vi "SimulateData.vi"(7 "DAQ":T1={"Data"={"Live"={"t0"=timestamp(0 s since 1904-01-01), "dt"=1.0, "Y"=[]}, "Accumulated"={"t0"=timestamp(0 s since 1904-01-01), "dt"=1.0, "Y"=[]}, "Averaged"={"t0"=timestamp(0 s since 1904-01-01), "dt"=1.0, "Y"=[]}, "data array"=[], "live time array"=[], "Live (decimated)"={"t0"=timestamp(0 s since 1904-01-01), "dt"=1.0, "Y"=[]}}, "Config"={"Input Config"=0, "Card"=enum."USB-6211", "100% Reflectance Standard (V)"=0.0, "Input Channel"="", "Average number of points"=0.0, "Trigger Level (V)"=0.0, "Rate (Hz)"=0, "End Time (s)"=0.0}, "Indicators"={"Final number of points"=0.0, "Number of samples"=0.0, "dt"=0.0, "Shots"=10, "Shot counter"=10, "Test counter"=10, "Background level (V)"=0.0, "DAQ task"="", "timestamp of data"=timestamp(0 s since 1904-01-01), "Test Type"=enum."A-Test"}} {"Config"."Input Config" items=["default"=-1, "RSE"=10083, "NRSE"=10078, "Differential"=10106, "Pseudodifferential"=12529]}, 8 "error in (no error)":errorcluster) -> (0 "error out":errorcluster, 5 "DAQ out":T1={"Data"={"Live"={"t0"=timestamp(0 s since 1904-01-01), "dt"=1.0, "Y"=[]}, "Accumulated"={"t0"=timestamp(0 s since 1904-01-01), "dt"=1.0, "Y"=[]}, "Averaged"={"t0"=timestamp(0 s since 1904-01-01), "dt"=1.0, "Y"=[]}, "data array"=[], "live time array"=[], "Live (decimated)"={"t0"=timestamp(0 s since 1904-01-01), "dt"=1.0, "Y"=[]}}, "Config"={"Input Config"=0, "Card"=enum."USB-6211", "100% Reflectance Standard (V)"=0.0, "Input Channel"="", "Average number of points"=0.0, "Trigger Level (V)"=0.0, "Rate (Hz)"=0, "End Time (s)"=0.0}, "Indicators"={"Final number of points"=0.0, "Number of samples"=0.0, "dt"=0.0, "Shots"=10, "Shot counter"=10, "Test counter"=10, "Background level (V)"=0.0, "DAQ task"="", "timestamp of data"=timestamp(0 s since 1904-01-01), "Test Type"=enum."A-Test"}} {"Config"."Input Config" items=["default"=-1, "RSE"=10083, "NRSE"=10078, "Differential"=10106, "Pseudodifferential"=12529]})   [LabVIEW 2017, in "DAQ.lvlib"]
uses:
  DAQ.lvlib
  Controls/Params.ctl
  Controls/DAQ Config.ctl
  Controls/DAQ Indicators.ctl
  System Control/CTLs/Test Type.ctl
  System Control/Main controller.lvlib
panel:
  out "Waveform Chart":waveform(dbl)(graph)
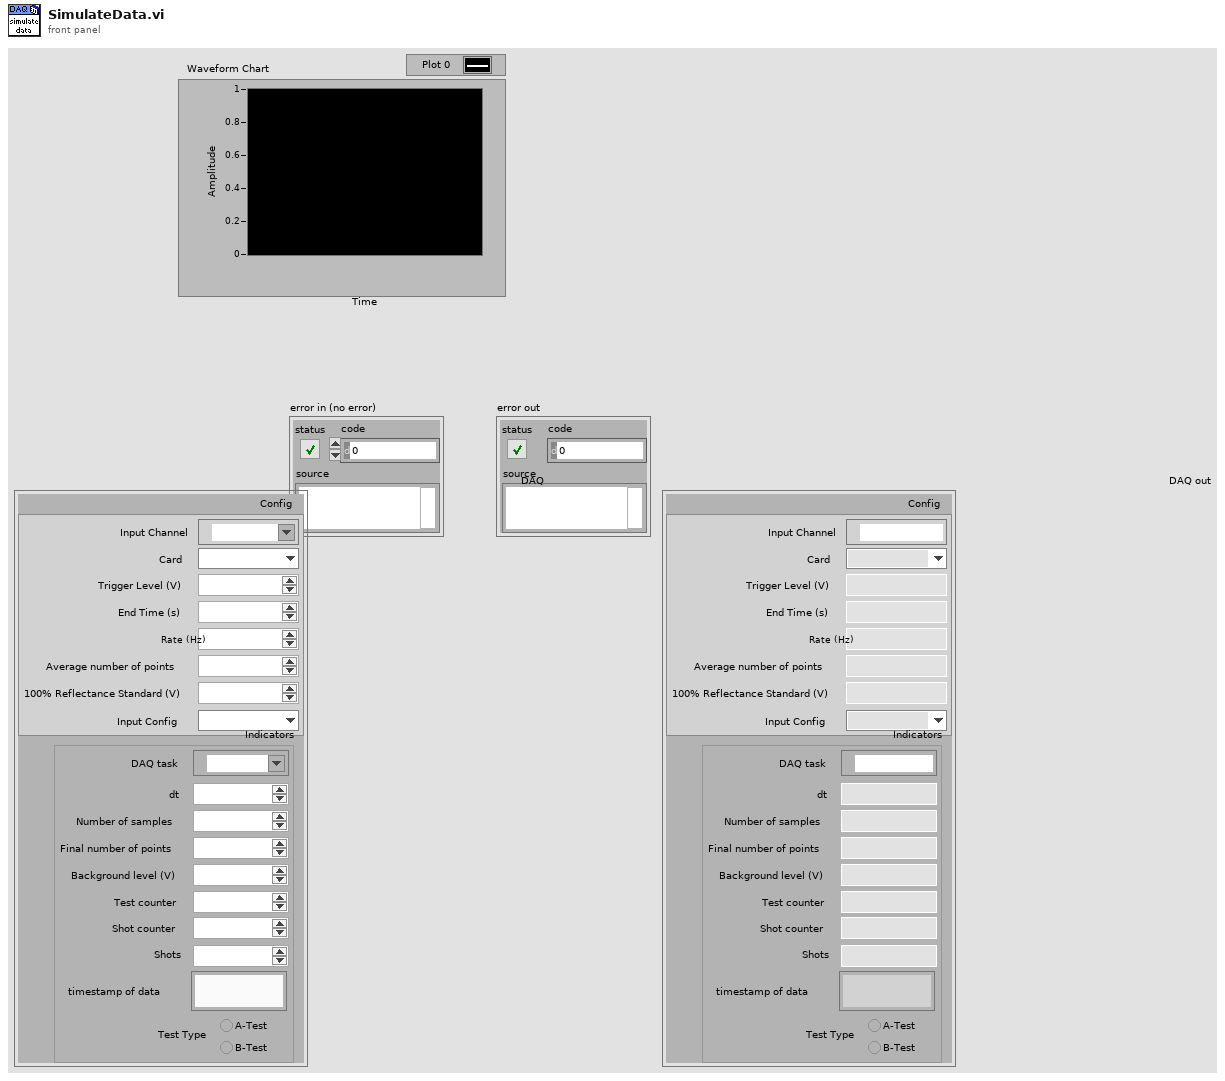
[diagram p1: front panel]
types:
  T1 = typedef "DAQ.lvlib/Params.ctl" = cluster{"Data":cluster{"Live":waveform(dbl), "Accumulated":waveform(dbl), "Averaged":waveform(dbl), "data array":dbl[], "live time array":dbl[], "Live (decimated)":waveform(dbl)}, "Config":T2, "Indicators":T3}
  T2 = typedef "DAQ.lvlib/DAQ Config.ctl" = cluster{"Input Config":i32, "Card":enum16{"USB-6211", "USB-6251", "USB-6361"}, "100% Reflectance Standard (V)":dbl, "Input Channel":tag, "Average number of points":dbl, "Trigger Level (V)":dbl, "Rate (Hz)":i32, "End Time (s)":dbl}
  T3 = typedef "DAQ.lvlib/DAQ Indicators.ctl" = cluster{"Final number of points":dbl, "Number of samples":dbl, "dt":dbl, "Shots":i32, "Shot counter":i32, "Test counter":i32, "Background level (V)":dbl, "DAQ task":refnum<k21>, "timestamp of data":timestamp, "Test Type":T4}
  T4 = typedef "Main controller.lvlib/Test Type.ctl" = enum32{"A-Test", "B-Test"}
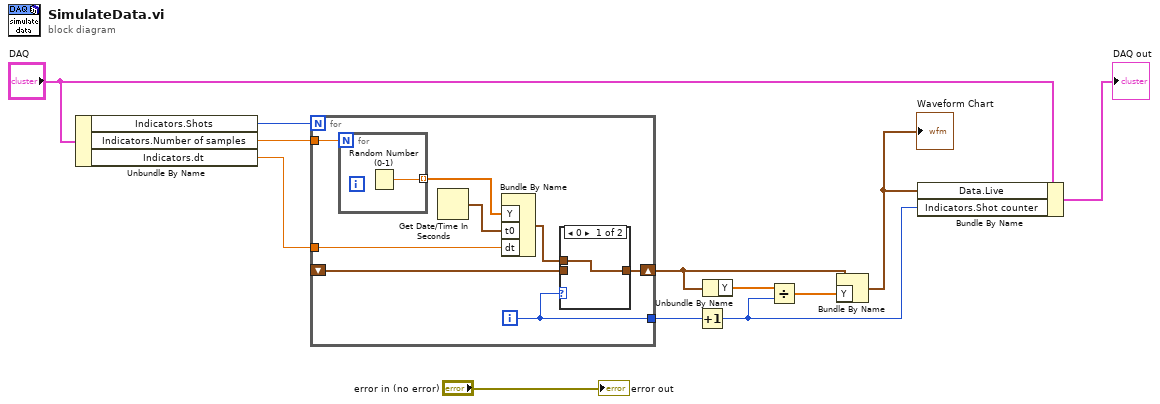
[diagram p0: block diagram]
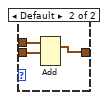
[diagram p2: hidden frame]
diagram:
  n1 = Unbundle By Name("DAQ") -> ("Indicators.Shots"=w9:i32, "Indicators.Number of samples"=w1:dbl, "Indicators.dt"=w2:dbl)
  n2 = for {
    N: w9 -> [_]
    tunnel: w1 -> [w20]
    tunnel: w2 -> [w17]
    shift-right: [w14] -> w4
    shift-left: _ -> [w15]
    tunnel: [w13] -> w3
    i -> [w13]
    n3 = for {
      N: w20 -> [_]
      tunnel: [w25] -> w18 mode=indexing
      n4 = Random Number (0-1)() -> (number: 0 to 1=w25:dbl)
    }
    n5 = Get Date/Time In Seconds() -> (seconds since 1Jan1904=w19:timestamp)
    n6 = Bundle By Name("Y"=w18, "t0"=w19, "dt"=w17) -> (w16:waveform(dbl))  [unwired: 1 in]
    n7 = case shown="0" w13 {
      tunnel: w16 -> [w21 w24]
      tunnel: w15 -> [_ w23]
      tunnel: [w21 w22] -> w14
      frame 0 {
      }
      frame Default {
        n8 = Add(1:w23, 2:w24) -> (0:w22:waveform(dbl))  [unwired: 1 in, 1 out]
      }
    }
  }
  n9 = Increment(x=w3) -> (x+1=w7:i32)
  n10 = Unbundle By Name(w4) -> ("Y"=w6:dbl[])
  n11 = Divide(x=w6, y=w7) -> (x/y=w5:dbl[])
  n12 = Bundle By Name(cluster=w4, "Y"=w5) -> (w10:waveform(dbl))
  "Waveform Chart" <- w10
  n13 = Bundle By Name(cluster="DAQ", "Data.Live"=w10, "Indicators.Shot counter"=w7) -> (→"DAQ out":T1)
  "error out" <- "error in (no error)"
